vi "Profile_Position_Mode.vi"() -> ()   [LabVIEW 2014]
panel:
  in  "stop":bool
  in  "1st RxPDO Mapping-TargetVelocity":i32
  in  "1st RxPDO Mapping-TargetPosition":i32
  out "error out":errorcluster
  # "6060h:\n\n0: Reserved\n1: Profile Position Mode\n3: Profile Velocity Mode\n4: Profile Torque Mode\n6: Homing Mode\n7: Interpolated Position Mode\n8: Cyclic Synchronous Position Mode\n9: Cyclic Synchronous Velocity Mode\n10: Cyclic Synchronous Torque Mode"
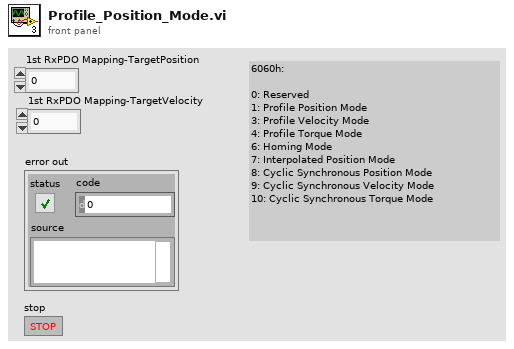
[diagram p1: front panel]
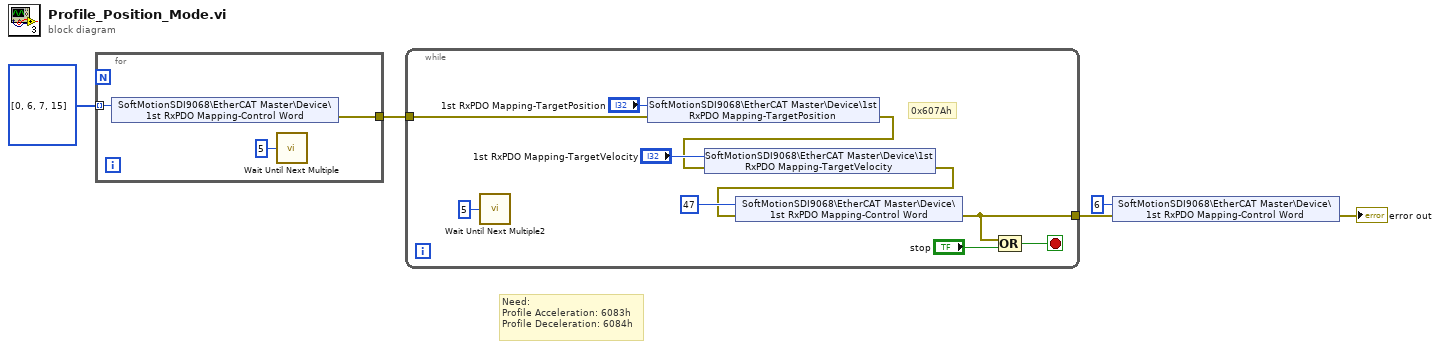
[diagram p0: block diagram]
diagram:
  # "Need:\nProfile Acceleration: 6083h\nProfile Deceleration: 6084h"
  n1 = for {
    tunnel: u16[] [0, 6, 7, 15] -> [w8] mode=indexing
    tunnel: [w6] -> w2
    n2 = shared-variable "SoftMotionSDI9068\\EtherCAT Master\\Device\\1st RxPDO Mapping-Control Word"(w8) -> (error out=w6:errorcluster)  [unwired: 1 in]
    n3 = call "Wait Until Next Multiple"("Count(mSec)"=u32 5) -> ()  [unwired: 1 out]
  }
  n4 = while {
    tunnel: w2 -> [w13]
    tunnel: [w9] -> w1
    stop <- w10 stop-if-true
    # "0x607Ah"
    n5 = call "Wait Until Next Multiple2"("Count(mSec)"=u32 5) -> ()  [unwired: 1 out]
    n6 = shared-variable "SoftMotionSDI9068\\EtherCAT Master\\Device\\1st RxPDO Mapping-TargetPosition"("1st RxPDO Mapping-TargetPosition", error in=w13) -> (error out=w12:errorcluster)
    n7 = shared-variable "SoftMotionSDI9068\\EtherCAT Master\\Device\\1st RxPDO Mapping-TargetVelocity"("1st RxPDO Mapping-TargetVelocity", error in=w12) -> (error out=w11:errorcluster)
    n8 = shared-variable "SoftMotionSDI9068\\EtherCAT Master\\Device\\1st RxPDO Mapping-Control Word"(u16 47 ("1st RxPDO Mapping-Control Word"), error in=w11) -> (error out=w9:errorcluster)
    n9 = Compound Arithmetic op=OR(w9, "stop") -> (w10:bool)
  }
  n10 = shared-variable "SoftMotionSDI9068\\EtherCAT Master\\Device\\1st RxPDO Mapping-Control Word"(u16 6 ("1st RxPDO Mapping-Control Word"), error in=w1) -> (error out=→"error out":errorcluster)
